vi "isNull.vi"(8 "error in (no error)":errorcluster, 11 "AbstractCustomer in":refnum<class "AbstractCustomer.lvclass">) -> (0 "error out":errorcluster, 2 "IsNull?":bool, 3 "AbstractCustomer out":refnum<class "AbstractCustomer.lvclass">)   [LabVIEW 2017, in "AbstractCustomer.lvclass"]
uses:
  AbstractCustomer.lvclass
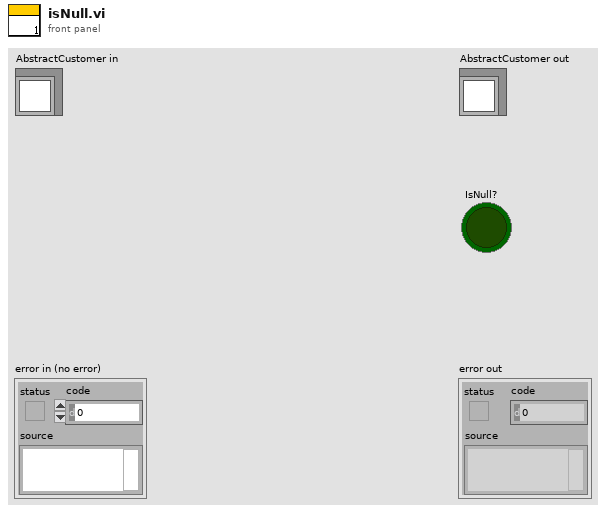
[diagram p1: front panel]
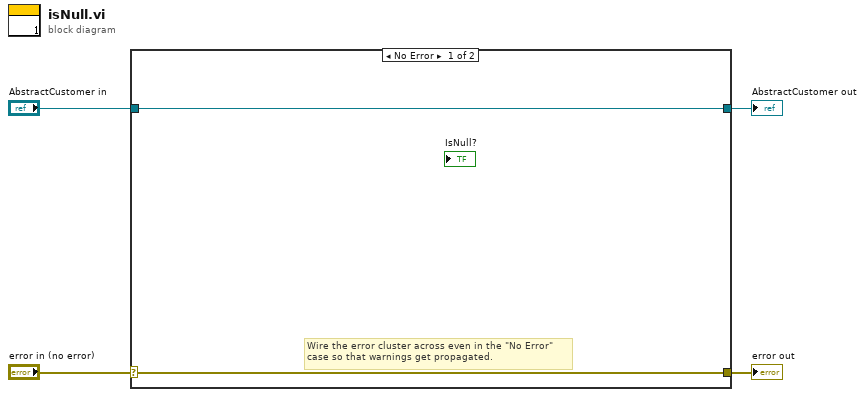
[diagram p0: block diagram]
diagram:
  n1 = case shown="No Error" "error in (no error)" {
    selector: "error in (no error)" -> [w5 w8]
    tunnel: [w5 w8] -> w3
    tunnel: [w6 w7] -> w1
    tunnel: "AbstractCustomer in" -> [w6 w7]
    frame No Error {
      # "Wire the error cluster across even in the \"No Error\"\ncase so that warnings get propagated."
    }
    frame Error {
    }
  }
  "error out" <- w3
  "AbstractCustomer out" <- w1
